vi "Control Target 2 Target Array.vi"(10 "Current Target":T3[](array[typedef])) -> (2 "Target  Array":T1[](array[typedef]))   [LabVIEW 2009]
uses:
  Target Data.ctl
  Data Access Objects/Metadata/LBCB Space.ctl
  Target.ctl
  Data Access Objects/Metadata/LBCB Number.ctl
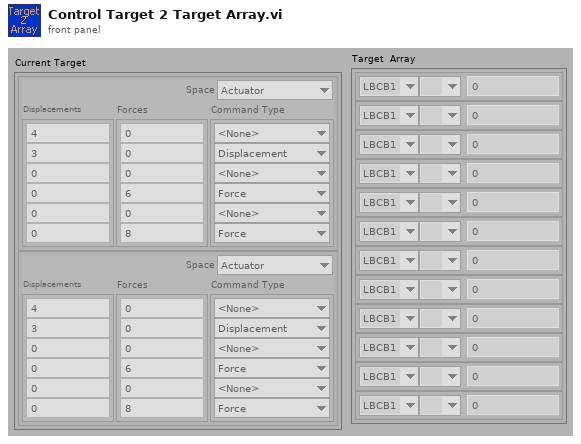
[diagram p1: front panel]
types:
  T1 = typedef "Target.ctl" = cluster{"LBCB Number":T2, "DOF Vectors":enum16{" ", "Dx", "Dy", "Dz", "Rx", "Ry", "Rz", "Fx", "Fy", "Fz", "Mx", "My", "Mz"}, "Amount":dbl}
  T2 = typedef "LBCB Number.ctl" = enum16{"LBCB1", "LBCB2"}
  T3 = typedef "Target Data.ctl" = cluster{"Displacements":dbl[], "Command Type":enum16{"<None>", "Displacement", "Force"}[], "Forces":dbl[], "Space":T4}
  T4 = typedef "LBCB Space.ctl" = enum16{"Actuator", "Cartesian"}
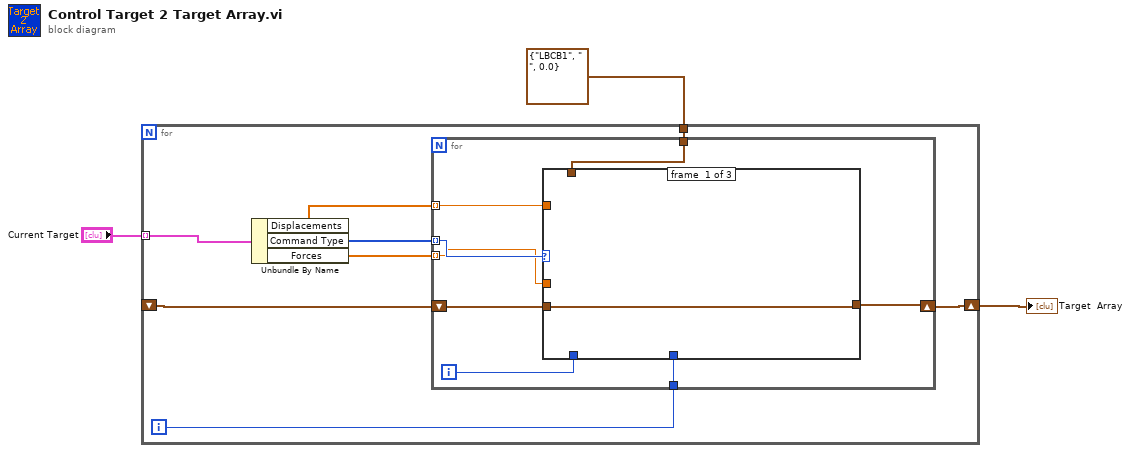
[diagram p0: block diagram]
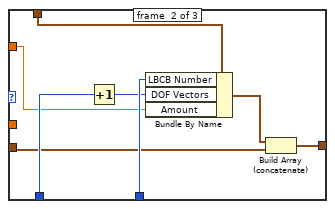
[diagram p2: hidden frame]
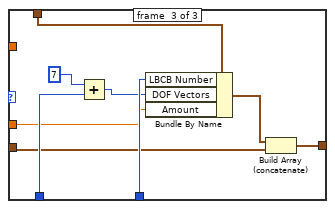
[diagram p3: hidden frame]
diagram:
  n1 = for {
    tunnel: "Current Target" -> [w11] mode=indexing
    tunnel: T1 {"LBCB Number"=enum."LBCB1", "DOF Vectors"=enum." ", "Amount"=0.0} ("Target") -> [w7]
    shift-right: [w4] -> w1
    shift-left: _ -> [w6]
    i -> [w5]
    n2 = Unbundle By Name(w11) -> ("Displacements"=w10:dbl[], "Command Type"=w9:enum16{"<None>", "Displacement", "Force"}[], "Forces"=w8:dbl[])
    n3 = for {
      tunnel: w10 -> [w18] mode=indexing
      tunnel: w9 -> [w19] mode=indexing
      tunnel: w8 -> [w17] mode=indexing
      shift-right: [w12] -> w4
      shift-left: w6 -> [w16]
      tunnel: w7 -> [w15]
      tunnel: w5 -> [w14]
      i -> [w13]
      n4 = case shown="\"Displacement\"" w19 {
        tunnel: w18 -> [_ w25 _]
        tunnel: w17 -> [_ _ w30]
        tunnel: w16 -> [w20 w22 w32]
        tunnel: w15 -> [_ w28 w37]
        tunnel: w14 -> [_ w27 w36]
        tunnel: w13 -> [_ w26 w35]
        tunnel: [w20 w23 w33] -> w12
        frame #0 {
        }
        frame #1 {
          n5 = Increment(x=w26) -> (x+1=w21:i32)
          n6 = Bundle By Name(cluster=w28, "LBCB Number"=w27, "DOF Vectors"=w21, "Amount"=w25) -> (w24:T1)
          n7 = Build Array (concatenate)(w24, w22) -> (w23:T1[])
        }
        frame #2 {
          n8 = Add(x=7, y=w35) -> (x+y=w29:i32)
          n9 = Bundle By Name(cluster=w37, "LBCB Number"=w36, "DOF Vectors"=w29, "Amount"=w30) -> (w34:T1)
          n10 = Build Array (concatenate)(w34, w32) -> (w33:T1[])
        }
      }
    }
  }
  "Target  Array" <- w1
